vi "Mars.vi"() -> ()   [LabVIEW 2012]
panel:
  in  "Target Ports":i32[](array[numeric])=[61540, 61542, 61544, 61546]
  in  "Transmission Ports":i32[](array[numeric])=[61541, 61543, 61545, 61547]
  in  "#Robots":i32=4
  out "Sending Ports?":bool
  out "Port Data Sent":string
  out "Error for all individual UDP":errorcluster
  out "UDP Robot Inputs & Status":T1(array[cluster])=[{"Left PWM"=1500, "Right PWM"=1500, "Robot Heading"=0, "UDP Transmitting Port"=61541, "UDP Receiving Port"=61540, "Robot Symbol"="R"}, {"Left PWM"=1500, "Right PWM"=1500, "Robot Heading"=0, "UDP Transmitting Port"=61543, "UDP Receiving Port"=61542, "Robot Symbol"="G"}, {"Left PWM"=1500, "Right PWM"=1500, "Robot Heading"=0, "UDP Transmitting Port"=61545, "UDP Receiving Port"=61544, "Robot Symbol"="B"}, {"Left PWM"=1500, "Right PWM"=1500, "Robot Heading"=0, "UDP Transmitting Port"=0, "UDP Receiving Port"=0, "Robot Symbol"="P"}]
  in  "#Targets":i32=5
  in  "Select Robot Control":string(combo)="Random Walk"
  in  "Wake On":bool
  out "error out":errorcluster
  out "Data sent":string
  out "Broadcasting?":bool
  in  "Position Array":i32[][](array[numeric])=[[200, 200], [200, 800], [800, 800], [800, 200], [500, 300], [895, 748], [330, 598], [300, 200], [350, 200]]
  in  "Target Names":string[](array[string])=["Q", "T", "U", "V", "W", "R", "G", "B", "P"]
  in  "Background Map":path=path "C:/Users/wwarner/Documents/S4/RobotX/robot-x/Forebrain/Magical World/Mars1.png"
  in  "Use Blank":bool=TRUE
  out "600 by 600 Picture Map":picture
  in  "STOP":bool
  # "Base Station UDP Broadcast"
  # "Target #1"
  # "Target #2"
  # "Target #3"
  # "Target #4"
  # "Target #5"
  # "Red Robot"
  # "Green Robot"
  # "Blue Robot"
  # "Purple Robot"
  # "Robots: Red, Green, Blue, (Purple)\nTargets: Pink"
  # "S: System Time"
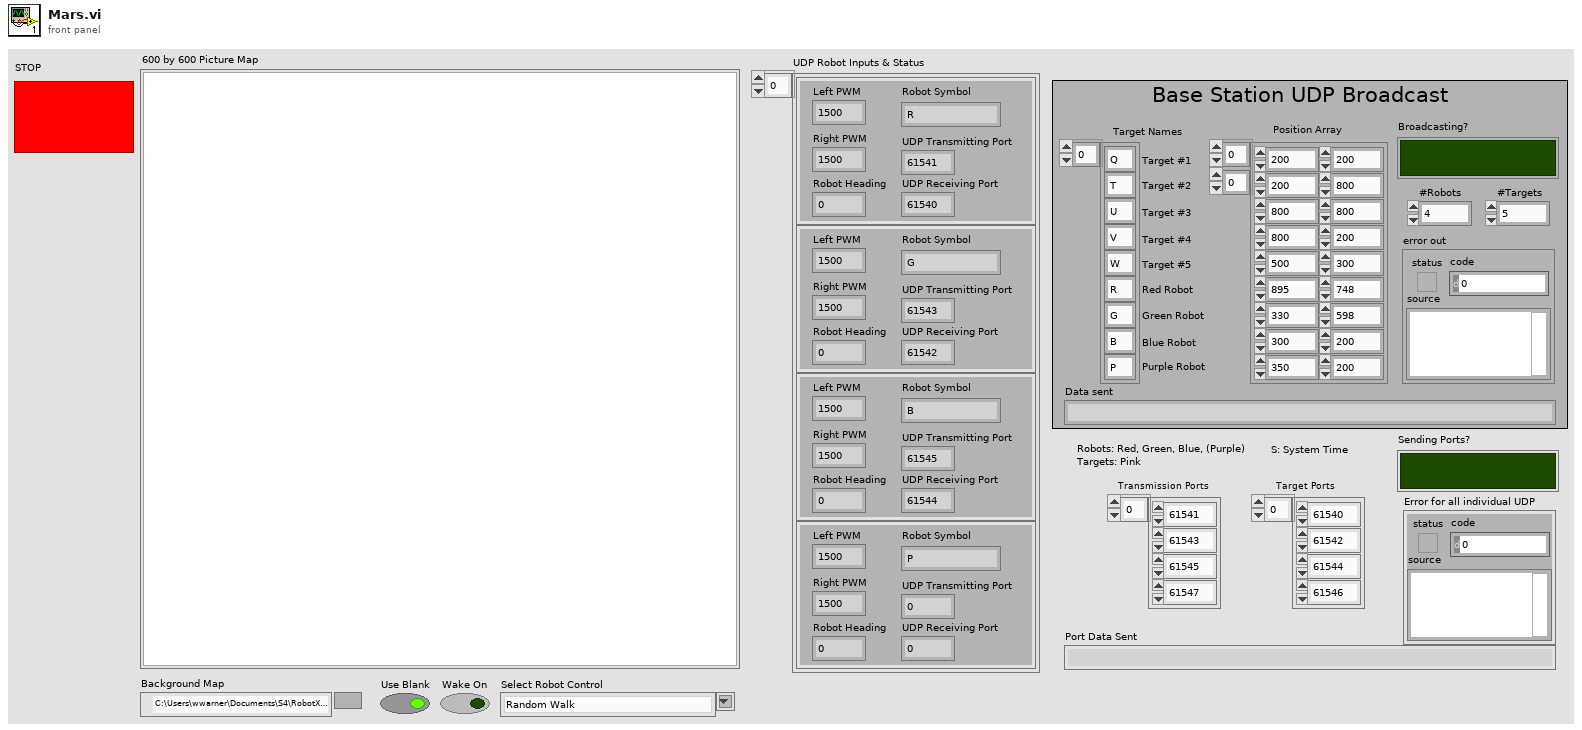
[diagram p1: front panel]
types:
  T1 = cluster{"Left PWM":i32, "Right PWM":i32, "Robot Heading":i32, "UDP Transmitting Port":i32, "UDP Receiving Port":i32, "Robot Symbol":string}[]
  T2 = typedef "LVBoundsTypeDef.ctl" = cluster{"Width":u32, "Height":u32}
  T3 = typedef "imagedata.ctl" = cluster{"image type":i32, "image depth":i32, "image":u8[], "mask":u8[], "colors":u32[], "Rectangle":cluster{"left":i16, "top":i16, "right":i16, "bottom":i16}}
  T4 = cluster{"Left PWM":i32, "Right PWM":i32, "Robot Heading":i32, "UDP Transmitting Port":i32, "UDP Receiving Port":i32, "Robot Symbol":string}
  T5 = cluster{"Position Array":i32[][], "Target Names":string[]}
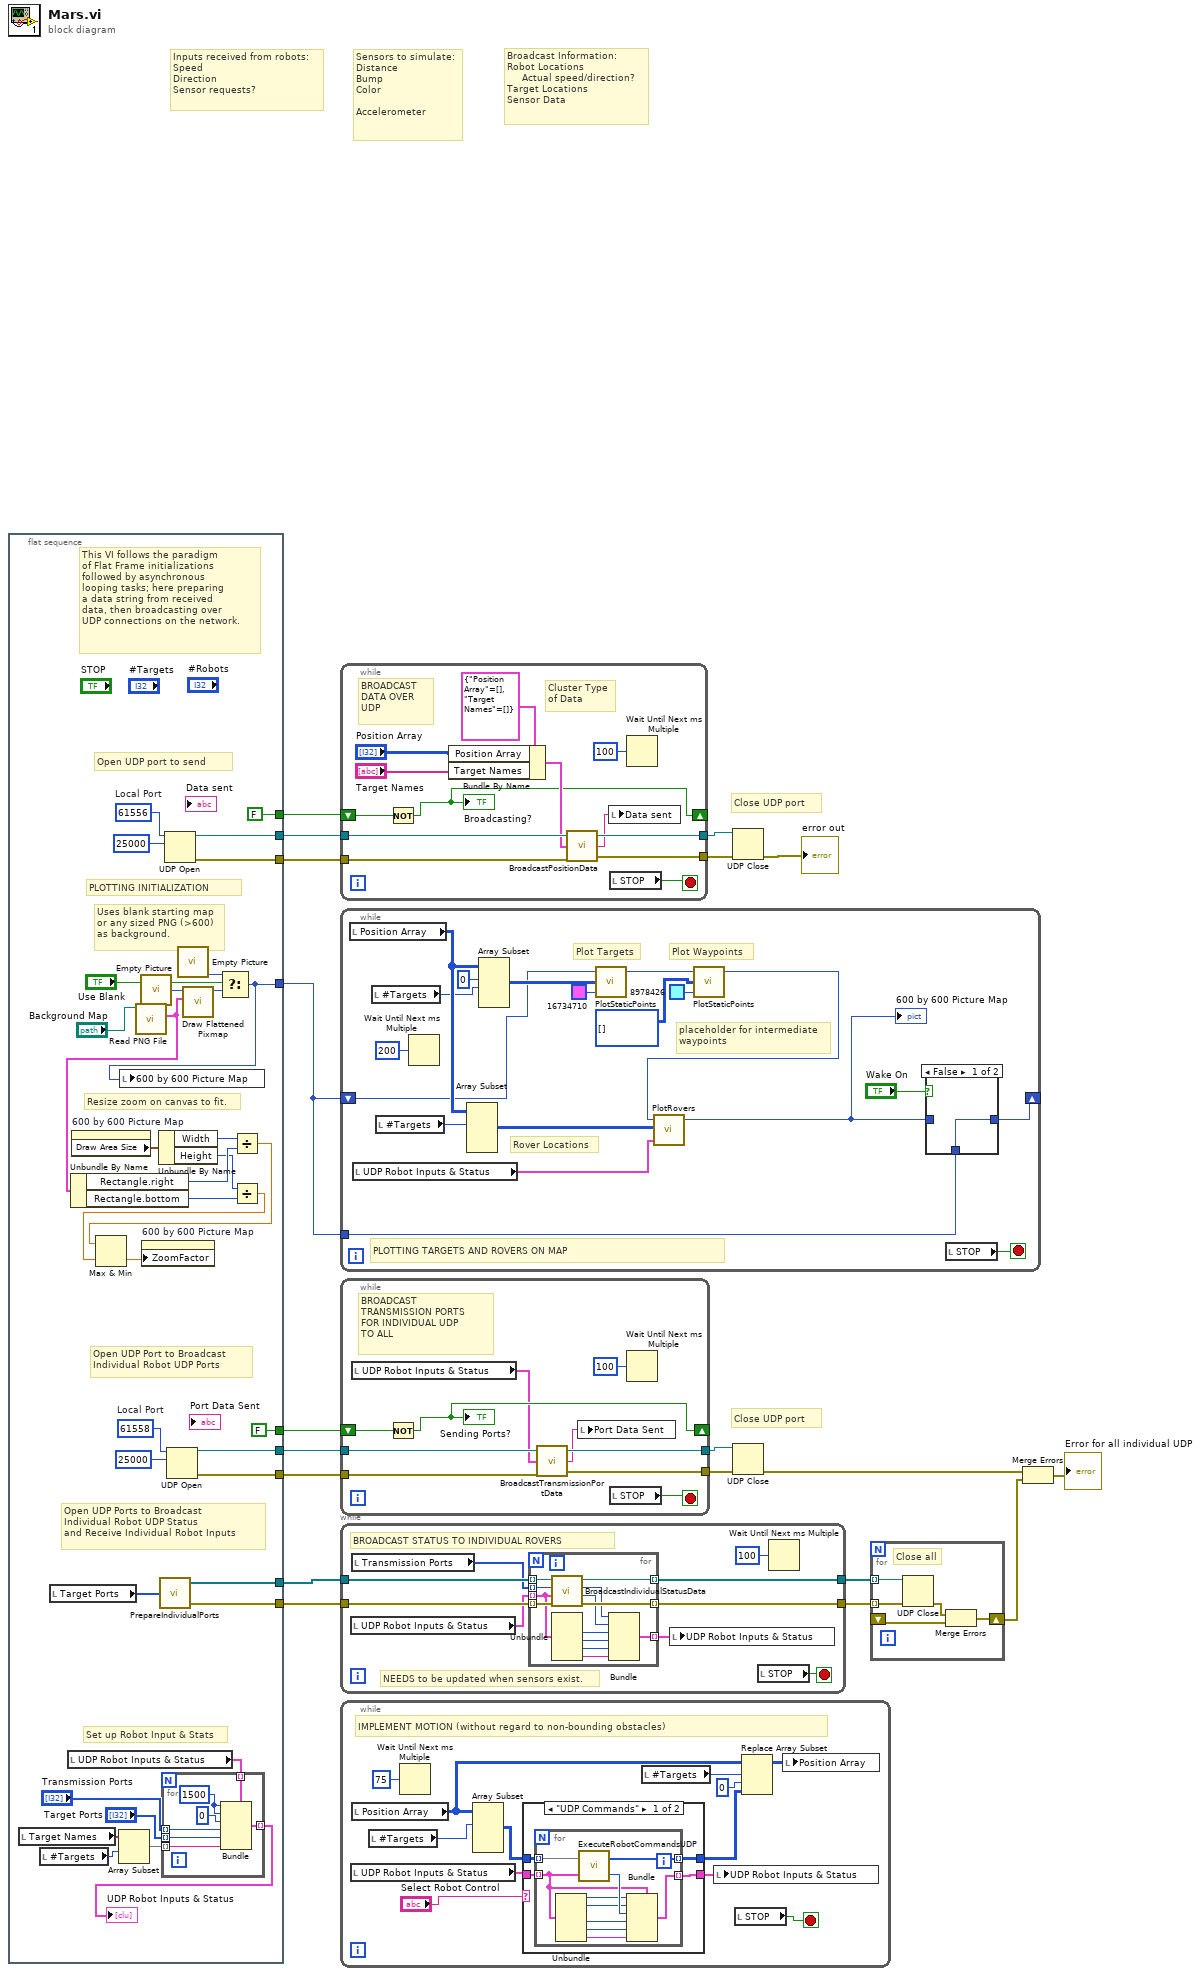
[diagram p0: block diagram]
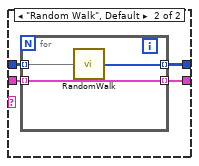
[diagram p3: hidden frame]
diagram:
  # "Close UDP port"
  # "Close UDP port"
  # "Broadcast Information:\nRobot Locations\n     Actual speed/direction?\nTarget Locations\nSensor Data"
  # "Sensors to simulate:\nDistance\nBump\nColor\n\nAccelerometer"
  # "Inputs received from robots:\nSpeed\nDirection\nSensor requests?"
  n1 = flat-sequence {
    tunnel: [w52] -> w14
    tunnel: [w51] -> w13
    tunnel: [FALSE] -> w16
    tunnel: [w44] -> w15
    tunnel: [w32] -> w10
    tunnel: [w31] -> w9
    tunnel: [FALSE] -> w8
    tunnel: [w21] -> w5
    tunnel: [w20] -> w4
    frame #0 {
      w33 = u16 61558  # Local Port
      w54 = u16 61556  # Local Port
      # "Open UDP Ports to Broadcast\nIndividual Robot UDP Status\nand Receive Individual Robot Inputs"
      # "Set up Robot Input & Stats"
      # "Open UDP Port to Broadcast\nIndividual Robot UDP Ports"
      # "PLOTTING INITIALIZATION"
      # "Resize zoom on canvas to fit."
      # "Uses blank starting map\nor any sized PNG (>600)\nas background."
      # "This VI follows the paradigm\nof Flat Frame initializations\nfollowed by asynchronous\nlooping tasks; here preparing\na data string from received\ndata, then broadcasting over\nUDP connections on the network."
      # "Open UDP port to send"
      n2 = local read "Target Names"() -> (w24:string[])
      n3 = local read "#Targets"() -> (w23:i32)
      n4 = local read "Target Ports"() -> (w22:i32[])
      n5 = local read "UDP Robot Inputs & Status"() -> (w26:T1)
      n6 = property on="600 by 600 Picture Map" class="Pict"() -> ("Draw Area Size"=w43:T2)  [unwired: 2 in, 2 out]
      n7 = Array Subset(array=w24, index=w23) -> (w29:string[])  [unwired: 1 in]
      n8 = call <vilib>:"Read PNG File.vi"("path to PNG file"="Background Map") -> ("image data"=w42:T3)  [unwired: 8 in, 2 out]
      n9 = Unbundle By Name(w42) -> ("Rectangle.right"=w40:i16, "Rectangle.bottom"=w38:i16)
      n10 = call "Empty Picture"() -> ("empty picture"=w47:picture)
      n11 = Unbundle By Name(w43) -> ("Width"=w41:u32, "Height"=w39:u32)
      n12 = call "PrepareIndividualPorts.vi"("Target Ports"=w22) -> ("Connection IDs"=w21:refnum<k16>[], "Error(s) Out"=w20:errorcluster[])  [unwired: 1 in]
      n13 = for {
        tunnel: [w61] -> w25 mode=indexing
        tunnel: w26 -> [w58] mode=indexing
        tunnel: "Transmission Ports" -> [w57] mode=indexing
        tunnel: "Target Ports" -> [w56] mode=indexing
        tunnel: w29 -> [w55] mode=indexing
        w60 = 1500 ("Right PWM")
        n14 = Bundle(cluster=w58, "Left PWM"=w60, "Right PWM"=w60, "Robot Heading"=0, "UDP Transmitting Port"=w57, "UDP Receiving Port"=w56, "Robot Symbol"=w55) -> (w61:T4)
      }
      "UDP Robot Inputs & Status" <- w25
      n15 = UDP Open(9:25000 ("timeout ms (25000)"), 11:w54) -> (port=w52:refnum<k16>, 0:w51:errorcluster)  [unwired: 1 in, 3 out]
      n16 = UDP Open(9:25000 ("timeout ms (25000)"), 11:w33) -> (port=w32:refnum<k16>, 0:w31:errorcluster)  [unwired: 1 in, 3 out]
      n17 = call "Empty Picture"() -> ("empty picture"=w45:picture)
      n18 = call <vilib>:"Draw Flattened Pixmap.vi"("image data"=w42, "picture"=w47) -> ("new picture"=w46:picture)  [unwired: 7 in]
      n19 = Select(t=w45, s="Use Blank", f=w46) -> (s? t:f=w44:picture)
      n20 = local write "600 by 600 Picture Map"(w44) -> ()
      n21 = Divide(x=w41, y=w40) -> (x/y=w36:dbl)
      n22 = Divide(x=w39, y=w38) -> (x/y=w35:dbl)
      n23 = Max & Min(x=w36, y=w35) -> (min(x,y)=w37:dbl)  [unwired: 1 out]
      n24 = property on="600 by 600 Picture Map" class="Pict"("ZoomFactor"=w37) -> ()  [unwired: 2 in, 2 out]
    }
  }
  n25 = while {
    tunnel: w14 -> [w71]
    tunnel: w13 -> [w70]
    tunnel: [w68] -> w18
    tunnel: [w67] -> w17
    shift-right: [w62] -> _
    shift-left: w16 -> [w63]
    stop <- w65 stop-if-true
    # "BROADCAST\nDATA OVER\nUDP"
    # "Cluster Type\nof Data"
    n26 = Not(x=w63) -> (.not. x?=w62:bool)
    "Broadcasting?" <- w62
    n27 = Bundle By Name(cluster=T5 {"Position Array"=[], "Target Names"=[]} ("Dummy Cluster"), "Position Array"="Position Array", "Target Names"="Target Names") -> (w69:T5)
    n28 = call "BroadcastPositionData.vi"("error in (no error)"=w70, "Simulated Satellite Data"=w69, "connection ID"=w71) -> ("error out"=w67:errorcluster, "Data sent"=w64:string, "connection ID out"=w68:refnum<k16>)
    n29 = local write "Data sent"(w64) -> ()
    n30 = local read "STOP"() -> (w65:bool)
    n31 = Wait Until Next ms Multiple(millisecond multiple=u32 100) -> ()  [unwired: 1 out]
  }
  n32 = while {
    shift-right: [w91] -> _
    shift-left: w15 -> [w83]
    tunnel: w15 -> [w87]
    stop <- w93 stop-if-true
    # "Rover Locations"
    # "placeholder for intermediate\nwaypoints"
    # "Plot Waypoints"
    # "Plot Targets"
    # "PLOTTING TARGETS AND ROVERS ON MAP"
    n33 = local read "Position Array"() -> (w88:i32[][])
    n34 = local read "UDP Robot Inputs & Status"() -> (w75:T1)
    n35 = local read "#Targets"() -> (w86:i32)
    n36 = local read "#Targets"() -> (w85:i32)
    n37 = Wait Until Next ms Multiple(millisecond multiple=u32 200) -> ()  [unwired: 1 out]
    n38 = Array Subset(array=w88, index (row)=w85) -> (w78:i32[][])  [unwired: 3 in]
    n39 = Array Subset(array=w88, index (row)=0 ("index"), length (row)=w86) -> (w84:i32[][])  [unwired: 2 in]
    n40 = call "PlotStaticPoints.vi"("Fill Color"=u32 16734710, "Position Array"=w84, "Picture In"=w83) -> ("Picture Out"=w81:picture)  [unwired: 2 in]
    n41 = call "PlotStaticPoints.vi"("Fill Color"=u32 8978426, "Position Array"=i32[][] [], "Picture In"=w81) -> ("Picture Out"=w77:picture)  [unwired: 2 in]
    n42 = call "PlotRovers.vi"("UDP Robot Inputs & Status"=w75, "Position Array"=w78, "Picture In"=w77) -> ("Picture Out"=w76:picture)  [unwired: 2 in]
    "600 by 600 Picture Map" <- w76
    n43 = case shown="False" "Wake On" {
      tunnel: w76 -> [_ w95]
      tunnel: [w94 w95] -> w91
      tunnel: w87 -> [w94 _]
      frame False {
      }
      frame True {
      }
    }
    n44 = local read "STOP"() -> (w93:bool)
  }
  n45 = while {
    tunnel: w10 -> [w105]
    tunnel: w9 -> [w104]
    tunnel: [w103] -> w12
    tunnel: [w102] -> w11
    shift-right: [w97] -> _
    shift-left: w8 -> [w98]
    stop <- w100 stop-if-true
    # "BROADCAST\nTRANSMISSION PORTS\nFOR INDIVIDUAL UDP\nTO ALL"
    n46 = local read "UDP Robot Inputs & Status"() -> (w96:T1)
    n47 = Not(x=w98) -> (.not. x?=w97:bool)
    "Sending Ports?" <- w97
    n48 = call "BroadcastTransmissionPortData.vi"("error in (no error)"=w104, "UDP Robot Inputs & Status"=w96, "connection ID"=w105) -> ("error out"=w102:errorcluster, "Data sent"=w99:string, "connection ID out"=w103:refnum<k16>)
    n49 = local write "Port Data Sent"(w99) -> ()
    n50 = local read "STOP"() -> (w100:bool)
    n51 = Wait Until Next ms Multiple(millisecond multiple=u32 100) -> ()  [unwired: 1 out]
  }
  n52 = while {
    tunnel: w5 -> [w111]
    tunnel: w4 -> [w110]
    tunnel: [w113] -> w3
    tunnel: [w112] -> w2
    stop <- w114 stop-if-true
    # "NEEDS to be updated when sensors exist."
    # "BROADCAST STATUS TO INDIVIDUAL ROVERS"
    n53 = local read "UDP Robot Inputs & Status"() -> (w109:T1)
    n54 = local read "Transmission Ports"() -> (w108:i32[])
    n55 = for {
      tunnel: [w127] -> w113 mode=indexing
      tunnel: [w126] -> w112 mode=indexing
      tunnel: w111 -> [w125] mode=indexing
      tunnel: w110 -> [w124] mode=indexing
      tunnel: w109 -> [w122] mode=indexing
      tunnel: w108 -> [w123] mode=indexing
      tunnel: [w115] -> w107 mode=indexing
      n56 = call "BroadcastIndividualStatusData.vi"("error in"=w124, "Robot Input & Status"=w122, "Transmission Port"=w123, "Connection ID"=w125) -> ("error out"=w126:errorcluster, "Right PWM"=w120:i32, "Left PWM"=w121:i32, "Connection ID"=w127:refnum<k16>)
      n57 = Unbundle(w122) -> ("Robot Heading"=w119:i32, "UDP Transmitting Port"=w118:i32, "UDP Receiving Port"=w117:i32, "Robot Symbol"=w116:string)  [unwired: 2 out]
      n58 = Bundle("Left PWM"=w121, "Right PWM"=w120, "Robot Heading"=w119, "UDP Transmitting Port"=w118, "UDP Receiving Port"=w117, "Robot Symbol"=w116) -> (w115:T4)  [unwired: 1 in]
    }
    n59 = local write "UDP Robot Inputs & Status"(w107) -> ()
    n60 = local read "STOP"() -> (w114:bool)
    n61 = Wait Until Next ms Multiple(millisecond multiple=u32 100) -> ()  [unwired: 1 out]
  }
  n62 = while {
    stop <- w139 stop-if-true
    # "IMPLEMENT MOTION (without regard to non-bounding obstacles)"
    n63 = local read "UDP Robot Inputs & Status"() -> (w128:T1)
    n64 = local read "Position Array"() -> (w137:i32[][])
    n65 = local read "#Targets"() -> (w135:i32)
    n66 = Wait Until Next ms Multiple(millisecond multiple=u32 75) -> ()  [unwired: 1 out]
    n67 = Array Subset(array=w137, index (row)=w135) -> (w133:i32[][])  [unwired: 3 in]
    n68 = case shown="\"UDP Commands\"" "Select Robot Control" {
      tunnel: w133 -> [w143 w157]
      tunnel: w128 -> [w142 w156]
      tunnel: [w141 w155] -> w130
      tunnel: [w140 w154] -> w129
      frame "UDP Commands" {
        n69 = for {
          tunnel: w143 -> [w153] mode=indexing
          tunnel: w142 -> [w149] mode=indexing
          tunnel: [w148] -> w141 mode=indexing
          tunnel: [w147] -> w140 mode=indexing
          n70 = Unbundle(w149) -> ("Left PWM"=w151:i32, "Right PWM"=w150:i32, "UDP Transmitting Port"=w146:i32, "UDP Receiving Port"=w145:i32, "Robot Symbol"=w144:string)  [unwired: 1 out]
          n71 = call "ExecuteRobotCommandsUDP.vi"("Robot Status"=w149, "Robot Position"=w153) -> ("Updated Robot Heading"=w152:i32, "Updated Robot Position"=w148:i32[])
          n72 = Bundle(cluster=w149, "Left PWM"=w151, "Right PWM"=w150, "Robot Heading"=w152, "UDP Transmitting Port"=w146, "UDP Receiving Port"=w145, "Robot Symbol"=w144) -> (w147:T4)
        }
      }
      frame "Random Walk", Default {
        n73 = for {
          tunnel: w157 -> [w160] mode=indexing
          tunnel: w156 -> [w158] mode=indexing
          tunnel: [w159] -> w155 mode=indexing
          tunnel: [w158] -> w154 mode=indexing
          n74 = call "RandomWalk.vi"("Current Robot Position"=w160) -> ("New Robot Position"=w159:i32[])
        }
      }
    }
    n75 = local read "#Targets"() -> (w134:i32)
    n76 = local write "UDP Robot Inputs & Status"(w129) -> ()
    n77 = local read "STOP"() -> (w139:bool)
    n78 = Replace Array Subset(array=w137, new element=w130, index (row)=w134, index (col)=0 ("disabled index (col)")) -> (w136:i32[][])
    n79 = local write "Position Array"(w136) -> ()
  }
  n80 = UDP Close(connection ID=w18, 8:w17) -> (error out=→"error out":errorcluster)  [unwired: 1 out]
  n81 = UDP Close(connection ID=w12, 8:w11) -> (error out=w6:errorcluster)  [unwired: 1 out]
  n82 = for {
    tunnel: w3 -> [w164] mode=indexing
    tunnel: w2 -> [w165] mode=indexing
    shift-right: [w162] -> w1
    shift-left: _ -> [w161]
    # "Close all"
    n83 = UDP Close(connection ID=w164, 8:w165) -> (error out=w163:errorcluster)  [unwired: 1 out]
    n84 = Merge Errors(w163, w161) -> (w162:errorcluster)
  }
  n85 = Merge Errors(w6, w1) -> (→"Error for all individual UDP":errorcluster)
